vi "Key Units.vi"(10 "Value":string, 11 "Key":string) -> (2 "Units":string, 3 "Variable Name":string, 5 "number":dbl)   [LabVIEW 2012, in "Design Server.lvlib"]
uses:
  Design Server.lvlib
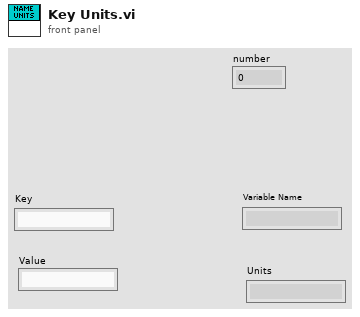
[diagram p1: front panel]
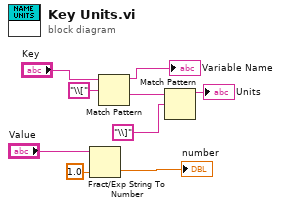
[diagram p0: block diagram]
diagram:
  n1 = Fract/Exp String To Number(string="Value", default (0 dbl)=1.0 ("default (0 DBL)")) -> (number=→"number":dbl)  [unwired: 2 in, 1 out]
  n2 = Match Pattern(string="Key", regular expression="\\[") -> (before substring=→"Variable Name":string, after substring=w6:string)  [unwired: 1 in, 2 out]
  n3 = Match Pattern(string=w6, regular expression="\\]") -> (before substring=→"Units":string)  [unwired: 1 in, 3 out]
